vi "H5_RefOpen.vi"(8 "error in (no error)":errorcluster, 10 "Filename":string, 11 "File Directory":path) -> (0 "error out":errorcluster, 2 "HDF5 Dataset Ref out":T1, 3 "HDF5 Ref out":T1, 5 "FilenameSimeStamped":string, 7 "FileDirectoryFinal":path)   [LabVIEW 2020]
uses:
  <vilib>/UPVI/lvhdf5/library.llb/HDF5 Ref.ctl
  <vilib>/UPVI/lvhdf5/file.llb/LVH5F Operation.ctl
  <vilib>/UPVI/lvhdf5/dataset.llb/LVH5D Operation.ctl
  <vilib>/Utility/miscctls.llb/LVRectTypeDef.ctl
  <vilib>/UPVI/lvhdf5/group.llb/H5G_obj_t.ctl
  <vilib>/UPVI/lvhdf5/utility.llb/Select HDF5 Dialog.vi
  <vilib>/UPVI/lvhdf5/utility.llb/Select HDF5 Dialog (Object Only).vi
  <vilib>/UPVI/lvhdf5/dataset.llb/Simple H5Dwrite (Variant).vi
  <vilib>/UPVI/lvhdf5/dataset.llb/Simple H5Dwrite.xnode
  <vilib>/UPVI/lvhdf5/file.llb/H5Fclose.vi
  <vilib>/UPVI/lvhdf5/identifier.llb/Not an HDF5 Refnum Constant.vi
  <vilib>/Utility/error.llb/Error Cluster From Error Code.vi
  <vilib>/UPVI/lvhdf5/dataset.llb/OpenCreateReplace Dataset by Element Type.vi
  <vilib>/UPVI/lvhdf5/dataspace.llb/H5Sselect_hyperslab.vi
  <vilib>/UPVI/lvhdf5/dataset.llb/H5Dwrite (Variant).vi
  <vilib>/UPVI/lvhdf5/dataset.llb/H5Dget_space.vi
  <vilib>/UPVI/lvhdf5/attribute.llb/private/LVH5AwriteWDTAttrs.vi
  <vilib>/UPVI/lvhdf5/dataspace.llb/H5Sclose.vi
  <vilib>/UPVI/lvhdf5/dataset.llb/H5Dclose.vi
  <vilib>/UPVI/lvhdf5/utility.llb/Select HDF5 Dialog (File and Object).vi
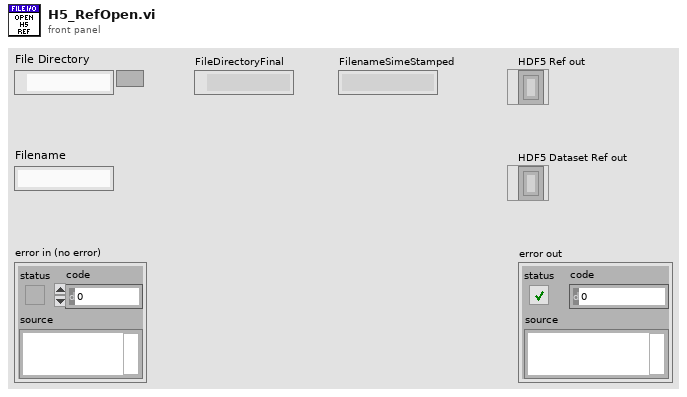
[diagram p1: front panel]
types:
  T1 = typedef "HDF5 Ref.ctl" = refnum<k1>
  T2 = typedef "LVH5D Operation.ctl" = enum16{"open", "replace", "create", "open or create", "create or replace", "create or replace with confirmation"}
  T3 = typedef "LVH5F Operation.ctl" = enum16{"open", "open or create", "create or replace", "create or replace (with confirmation)", "create", "open (read only)"}
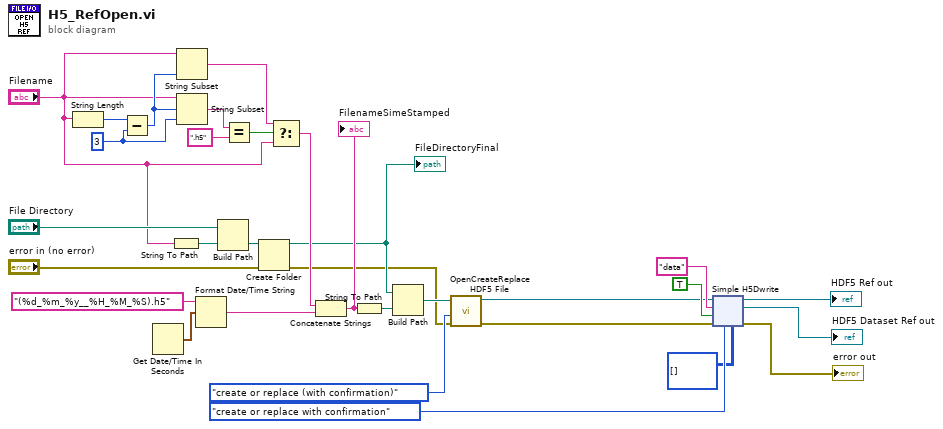
[diagram p0: block diagram]
diagram:
  w17 = 3 ("length (rest)")
  n1 = String Length(string="Filename") -> (length=w18:i32)
  n2 = Subtract(x=w18, y=w17) -> (x-y=w14:i32)
  n3 = Get Date/Time In Seconds() -> (seconds since 1Jan1904=w24:timestamp)
  n4 = String To Path(string="Filename") -> (path=w1:path)
  n5 = String Subset(string="Filename", length (rest)=w14) -> (substring=w12:string)  [unwired: 1 in]
  n6 = String Subset(string="Filename", offset (0)=w14, length (rest)=w17) -> (substring=w16:string)
  n7 = Format Date/Time String(time format string (%c)="(%d_%m_%y__%H_%M_%S).h5", seconds (now)=w24) -> (date/time string=w23:string)  [unwired: 1 in]
  n8 = Build Path(base path="File Directory", name or relative path=w1) -> (appended path=w8:path)
  n9 = Equal?(x=w16, y=".h5") -> (x = y?=w13:bool)
  n10 = Create Folder(path (use dialog)=w8, error in="error in (no error)") -> (created path=w5:path, error out=w3:errorcluster)  [unwired: 1 in, 1 out]
  "FileDirectoryFinal" <- w5
  n11 = Select(t=w12, s=w13, f="Filename") -> (s? t:f=w11:string)
  n12 = Concatenate Strings(w11, w23) -> (w26:string)
  "FilenameSimeStamped" <- w26
  n13 = String To Path(string=w26) -> (path=w6:path)
  n14 = Build Path(base path=w5, name or relative path=w6) -> (appended path=w22:path)
  n15 = call <vilib>:"OpenCreateReplace HDF5 File.vi"("error in (no error)"=w3, "function (open or create)"=LVH5F_Operation."create or replace (with confirmation)", "path"=w22) -> ("error out"=w10:errorcluster, "HDF5 Ref out"=w9:T1)  [unwired: 5 in]
  n16 = xnode "Simple H5Dwrite"("Dataset Path"="data", "Unlimited  dataset (F)"=TRUE, "error in (no error)"=w10, "operation (open or create)"=LVH5D_Operation."create or replace with confirmation", "HDF5 Path or Ref"=w9, "Data"=i16[][] [] ("Waveform")) -> ("HDF5 Dataset Ref out"=→"HDF5 Dataset Ref out":T1, "HDF5 Ref out"=→"HDF5 Ref out":T1, "error out"=→"error out":errorcluster)  [unwired: 2 in]
